vi "TEST_3DOF.vi"() -> ()   [LabVIEW 2013]
uses:
  <vilib>/Instr/_visa.llb/VISA Configure Serial Port (Instr).vi
panel:
  in  "대기 시간(ms)":u32=500
  out "숫자형":i32
  out "Read String":string
  out "Ethernet M":i32
  out "Ethernet R":i32
  out "Ethernet L":i32
  out "Ethernet Axis":string
  in  "포트":u16=50
  in  "IP":string="127.0.0.1"
  in  "NetON":bool
  out "Axis":string
  out "END":string
  in  "cutting":bool
  out "C":i32
  out "B":i32
  out "A":i32
  out "M":i32
  out "R":i32
  out "L":i32
  out "Serial Port Byte":u32=15188
  in  "WriteON":bool
  in  "정지":bool
  in  "baud rate (9600)":u32=2400 caption="보 전송속도(9600)"
  in  "VISA 리소스 이름":refnum<visa-resource-name>="COM3"
  in  "Write":string="L100nM100nR100nn"
  out "Read":string
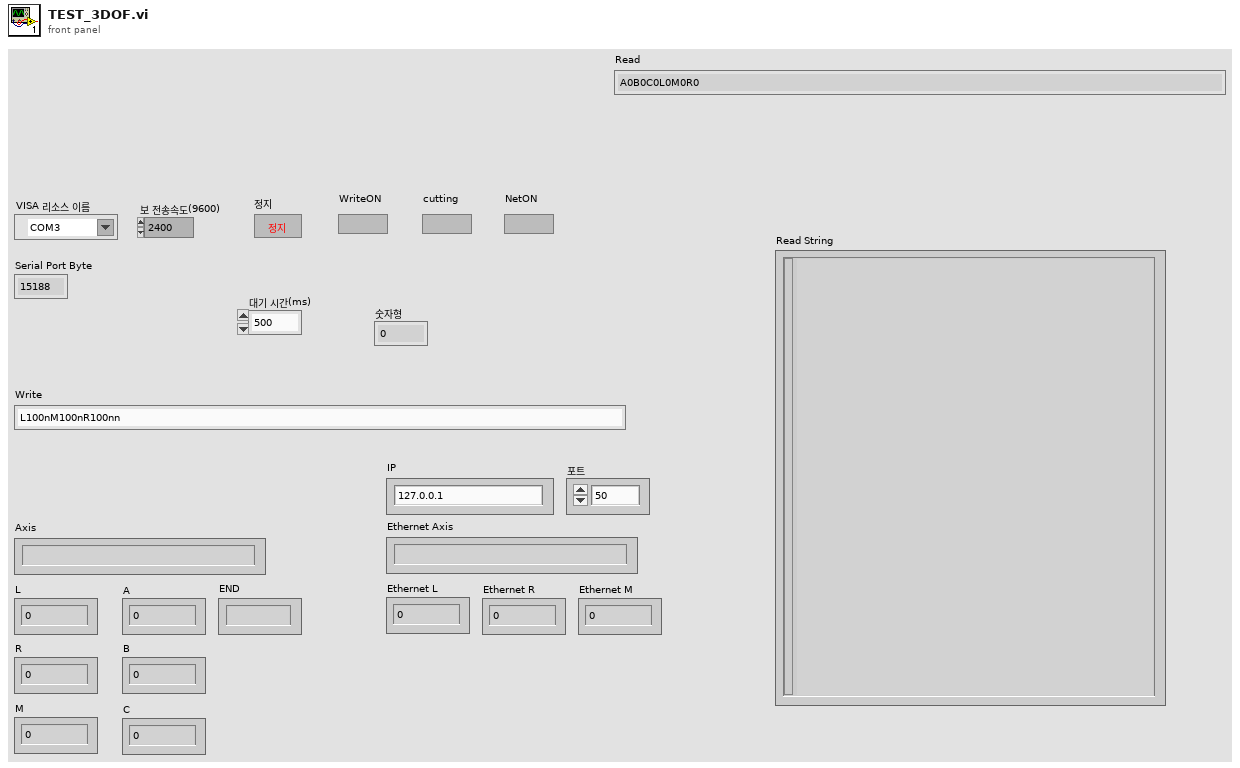
[diagram p1: front panel]
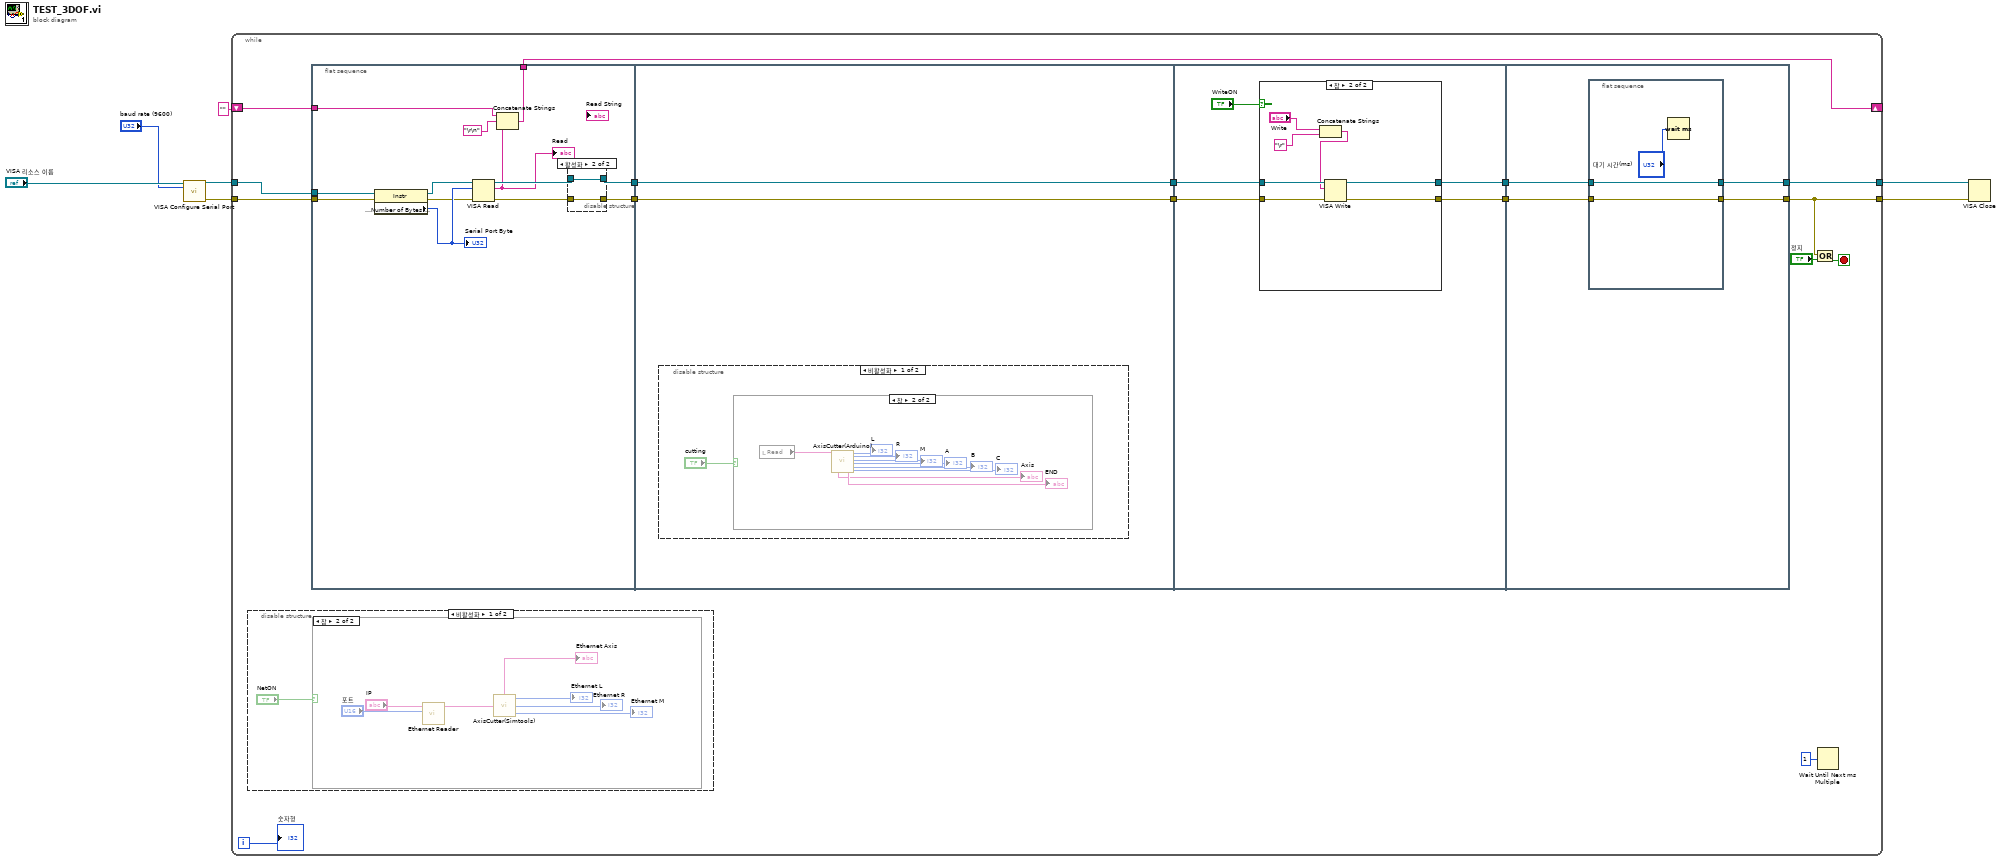
[diagram p0: block diagram]
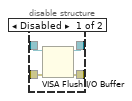
[diagram p4: hidden frame]
diagram:
  n1 = call-poly "VISA Configure Serial Port"("VISA resource name"="VISA 리소스 이름", "baud rate (9600)"="baud rate (9600)") -> ("VISA resource name out"=w6:refnum<visa-resource-name>, "error out"=w7:errorcluster)  [unwired: 12 in]
  n2 = while {
    tunnel: w7 -> [w15]
    tunnel: w6 -> [w16]
    tunnel: [w14] -> w3
    tunnel: [w10] -> w2
    shift-right: [w8] -> _
    shift-left: "" -> [w9]
    i -> [w12]
    stop <- w11 stop-if-true
    n3 = disable-structure shown="비활성화" {
      frame Disabled {
        n4 = case shown="참" "NetON" {
          frame False {
          }
          frame True {
            n5 = call "Ethernet Reader.vi"("IP"="IP", "포트"="포트") -> ("Axis"=w25:string)  [unwired: 6 in, 1 out]
            n6 = call "AxisCutter(Simtools).vi"("수신"=w25) -> ("Axis"=→"Ethernet Axis":string, "L"=→"Ethernet L":i32, "R"=→"Ethernet R":i32, "M"=→"Ethernet M":i32)
          }
        }
      }
      frame Enabled {
      }
    }
    n7 = flat-sequence {
      tunnel: [w36] -> w22
      tunnel: [w38] -> w21
      tunnel: w16 -> [w43]
      tunnel: w15 -> [w42]
      tunnel: w9 -> [w35]
      tunnel: [w32] -> w8
      tunnel: [w52] -> w20
      tunnel: w22 -> [w52]
      tunnel: [w51] -> w19
      tunnel: w21 -> [w51]
      tunnel: w20 -> [w66]
      tunnel: w19 -> [w65]
      tunnel: [w64] -> w18
      tunnel: [w63] -> w17
      tunnel: w18 -> [w80]
      tunnel: w17 -> [w79]
      tunnel: [w78] -> w14
      tunnel: [w77] -> w10
      frame #0 {
        n8 = property class="Instr"(reference=w43, error in=w42) -> (reference out=w40:refnum<visa-resource-name>, error out=w39:errorcluster, "Serial Settings:Number of Bytes at Serial Port"=w41:u32)
        "Serial Port Byte" <- w41
        n9 = VISA Read(VISA resource name=w40, byte count=w41, error in (no error)=w39) -> (VISA resource name out=w44:refnum<visa-resource-name>, read buffer=w33:string, error out=w37:errorcluster)  [unwired: 1 out]
        "Read" <- w33
        n10 = Concatenate Strings(w35, "\r\n", w33) -> (w32:string)
        n11 = disable-structure shown="활성화" {
          disable-tunnel: w44 -> [w48 w50]
          disable-tunnel: [w47 w50] -> w38
          disable-tunnel: w37 -> [w46 w49]
          disable-tunnel: [w45 w49] -> w36
          frame Disabled {
            n12 = VISA Flush I/O Buffer(VISA resource name=w48, error in (no error)=w46) -> (VISA resource name out=w47:refnum<visa-resource-name>, error out=w45:errorcluster)  [unwired: 1 in]
          }
          frame Enabled {
          }
        }
      }
      frame #1 {
        n13 = disable-structure shown="비활성화" {
          frame Disabled {
            n14 = case shown="참" "cutting" {
              frame False {
              }
              frame True {
                n15 = local read "Read"() -> (w54:string)
                n16 = call "AxisCutter(Arduino).vi"("수신"=w54) -> ("Axis"=→"Axis":string, "END"=→"END":string, "L"=→"L":i32, "R"=→"R":i32, "M"=→"M":i32, "A"=→"A":i32, "B"=→"B":i32, "C"=→"C":i32)  [unwired: 11 in]
              }
            }
          }
          frame Enabled {
          }
        }
      }
      frame #2 {
        n17 = case shown="참" "WriteON" {
          tunnel: w65 -> [w69 w76]
          tunnel: w66 -> [w68 w75]
          tunnel: [w69 w74] -> w64
          tunnel: [w68 w73] -> w63
          frame False {
          }
          frame True {
            n18 = Concatenate Strings("Write", "\r") -> (w70:string)
            n19 = VISA Write(VISA resource name=w76, write buffer=w70, error in (no error)=w75) -> (VISA resource name out=w74:refnum<visa-resource-name>, error out=w73:errorcluster)  [unwired: 1 out]
          }
        }
      }
      frame #3 {
        n20 = flat-sequence {
          tunnel: w80 -> [w83]
          tunnel: [w83] -> w78
          tunnel: [w82] -> w77
          tunnel: w79 -> [w82]
          frame #0 {
            n21 = Wait (ms)(milliseconds to wait="대기 시간(ms)") -> ()  [unwired: 1 out]
          }
        }
      }
    }
    n22 = Or(x=w10, y="정지") -> (x .or. y?=w11:bool)
    n23 = Wait Until Next ms Multiple(millisecond multiple=u32 1 ("ms 배수")) -> ()  [unwired: 1 out]
    "숫자형" <- w12
  }
  n24 = VISA Close(VISA resource name=w3, error in (no error)=w2) -> ()  [unwired: 1 out]
